vi "Test List Tags By Type.vi"() -> ()   [LabVIEW 2021]
uses:
  Source/Omni-Bus/Omni_Bus.lvclass
  Source/Aggregator Bus/Aggregator Bus.lvclass
  <vilib>/TSA/Abstract Data Classes/Constants/Support/Bool/Bool.vi
  <vilib>/TSA/Abstract Data Classes/Constants/Support/Bool/Const_Bool.lvclass
  <vilib>/TSA/Abstract Data Classes/Constants/Support/Str/Str.vi
  <vilib>/TSA/Abstract Data Classes/Constants/Support/Str/Const_Str.lvclass
  <vilib>/TSA/Abstract Data Classes/Constants/Support/DBL/DBL.vi
  <vilib>/TSA/Abstract Data Classes/Constants/Support/DBL/Const_DBL.lvclass
  <vilib>/TSA/Abstract Data Classes/Constants/Support/I32/I32.vi
  <vilib>/TSA/Abstract Data Classes/Constants/Support/I32/Const_I32.lvclass
  Source/Omni-Bus/Support/Broad Types.ctl
  <vilib>/TSA/Abstract Data Classes/Abs_Types/Boolean/Abs_Boolean.lvclass
  C:/Program Files (x86)/National Instruments/LabVIEW 2021/vi.lib/TSA/Abstract Data Classes/Abs_Types/Value/Abs_Value.lvclass
  C:/Program Files (x86)/National Instruments/LabVIEW 2021/vi.lib/TSA/Abstract Data Classes/Abs_Types/Type/Abs_Type.lvclass
  C:/Program Files (x86)/National Instruments/LabVIEW 2021/vi.lib/TSA/Abstract Data Classes/Abs_Types/Boolean/Abs_Boolean.lvclass
  C:/Program Files (x86)/National Instruments/LabVIEW 2021/vi.lib/TSA/Abstract Data Classes/Abs_Types/Double Float/Abs_Double Float.lvclass
  C:/Program Files (x86)/National Instruments/LabVIEW 2021/vi.lib/TSA/Abstract Data Classes/Abs_Types/Floating Point/Abs_Floating Point.lvclass
  C:/Program Files (x86)/National Instruments/LabVIEW 2021/vi.lib/TSA/Abstract Data Classes/Abs_Types/Numeric/Abs_Numeric.lvclass
  C:/Program Files (x86)/National Instruments/LabVIEW 2021/vi.lib/TSA/Abstract Data Classes/Constants/Support/DBL/Const_DBL.lvclass
  C:/Program Files (x86)/National Instruments/LabVIEW 2021/vi.lib/TSA/Abstract Data Classes/Constants/Support/Interface/Const_Intf.lvclass
  <vilib>/TSA/Abstract Data Classes/Abs_Types/String/Abs_String.lvclass
  C:/Program Files (x86)/National Instruments/LabVIEW 2021/vi.lib/TSA/Abstract Data Classes/Abs_Types/String/Abs_String.lvclass
  <vilib>/TSA/Abstract Data Classes/Abs_Types/I32 Integer/Abs_I32 Integer.lvclass
  C:/Program Files (x86)/National Instruments/LabVIEW 2021/vi.lib/TSA/Abstract Data Classes/Abs_Types/Integer/Abs_Integer.lvclass
  C:/Program Files (x86)/National Instruments/LabVIEW 2021/vi.lib/TSA/Abstract Data Classes/Abs_Types/I32 Integer/Abs_I32 Integer.lvclass
  <vilib>/TSA/Abstract Data Classes/Abs_Types/Value/Abs_Value.lvclass
  C:/Users/Tim/Documents/GitHub/Omni-Bus/Source/Omni-Bus/Bus Access/Bus_Access.lvclass
  C:/Users/Tim/Documents/GitHub/Omni-Bus/Source/Aggregator Bus/Aggregator Bus.lvclass
panel:
  out "Tags":string[](array[string])
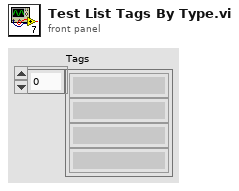
[diagram p1: front panel]
types:
  T1 = typedef "Omni_Bus.lvclass/Broad Types.ctl" = enum16{"All Tags", "NI Specific Type", "Boolean", "String", "Numeric", "Float", "Integer", "Collection", "All Value Types", "Non Value Types"}
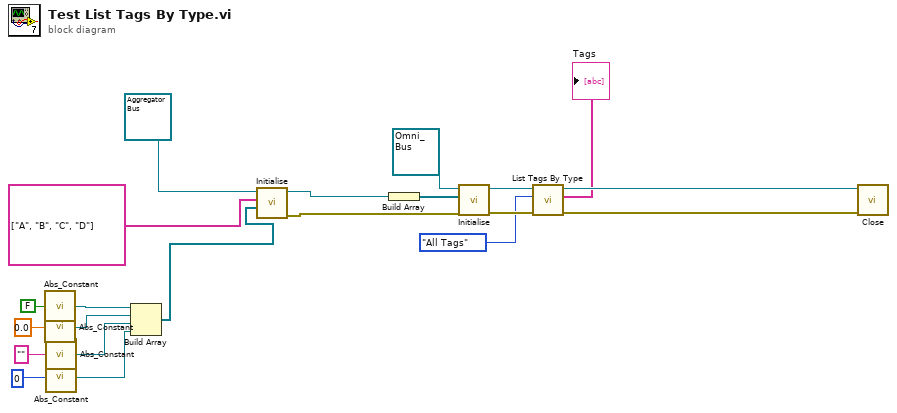
[diagram p0: block diagram]
diagram:
  n1 = call-poly <vilib>:"Abs_Constant.vi"("Boolean"=FALSE) -> ("Abs_Boolean.lvclass"=w19:refnum<class "Abs_Boolean.lvclass">)  [unwired: 4 in]
  n2 = call-poly <vilib>:"Abs_Constant.vi"("Value"=0.0) -> ("Constant"=w18:refnum<class "Const_DBL.lvclass">)  [unwired: 4 in]
  n3 = call-poly <vilib>:"Abs_Constant.vi"("String"="") -> ("Abs_String.lvclass"=w17:refnum<class "Abs_String.lvclass">)  [unwired: 4 in]
  n4 = call-poly <vilib>:"Abs_Constant.vi"("Value"=0) -> ("Constant"=w8:refnum<class "Abs_I32 Integer.lvclass">)  [unwired: 4 in]
  n5 = Build Array(w19, w18, w17, w8) -> (w1:refnum<class "Abs_Value.lvclass">[])
  n6 = call "Initialise.vi"("Values"=w1, "Tags"=string[] ["A", "B", "C", "D"], "Aggregator Bus in"=refnum<class "Aggregator Bus.lvclass"> refnum ("Data in")) -> ("error out"=w5:errorcluster, "Aggregator Bus out"=w4:refnum<class "Aggregator Bus.lvclass">)  [unwired: 7 in]
  n7 = Build Array(w4) -> (w20:refnum<class "Aggregator Bus.lvclass">[])
  n8 = call-dynamic "Initialise.vi"("error in (no error)"=w5, "Bus Access"=w20, "Var Bus in"=refnum<class "Omni_Bus.lvclass"> refnum) -> ("error out"=w13:errorcluster, "Var Bus out"=w14:refnum<class "Omni_Bus.lvclass">)  [unwired: 7 in]
  n9 = call "List Tags By Type.vi"("error in (no error)"=w13, "Broad Types"=Broad_Types."All Tags", "Var Bus in"=w14) -> ("error out"=w11:errorcluster, "Tags"=→"Tags":string[], "Var Bus out"=w12:refnum<class "Omni_Bus.lvclass">)  [unwired: 5 in, 1 out]
  n10 = call-dynamic "Close.vi"("error in (no error)"=w11, "Data in"=w12) -> ()  [unwired: 8 in, 2 out]
